vi "Transfer.vi"(7 "Timeout":i32 format="%d ms", 8 "error in":errorcluster, 9 "Parameters":T2 {"Data" format="%02x"; "Multiplexer"."Sub Index" format="%02x"; "Multiplexer"."Index" format="%04x"}, 10 "SDO Transfer":refnum<class "SDO Transfer.lvclass">, 11 "SDO Manager in":refnum<class "SDO Manager.lvclass">) -> (0 "error out":errorcluster, 3 "SDO Result":T3 {"SDO abort code"."Value" items=["Toggle bit not allowed"=84082688, "SDO protocol timed out"=84148224, "Client/server command specifier not valid or unknown"=84148225, "Invalid block size (block mode only)"=84148226, "Invalid sequence number (block mode only)"=84148227, "CRC error (block mode only)"=84148228, "Out of memory"=84148229, "Attempt to read a write only object"=100728833, "Attempt to write a read only object"=100728834, "Object does not exist in the object dictionary"=100794368, "Object cannot be mapped to the PDO"=100925505, "The number and length of the objects to be mapped would exceed PDO length"=100925506, "General parameter incompatibility reason"=100925507, "General internal incompatibility in the device"=100925511, "Access failed due to an hardware error"=101056512, "Data type does not match, length of service parameter does not match"=101122064, "Data type does not match, length of service parameter too high"=101122066, "Data type does not match, length of service parameter too low"=101122067, "Sub-index does not exist"=101253137, "Invalid value for parameter (download only)"=101253168, "Value of parameter written too high (download only)"=101253169, "Value of parameter written too low (download only)"=101253170, "Maximum value is less than minimum value"=101253174, "Resource not available: SDO connection"=101318691, "General error"=134217728, "Data cannot be transferred or stored to the application"=134217760, "Data cannot be transferred or stored to the application because of local control"=134217761, "Data cannot be transferred or stored to the application because of the present device stable"=134217762, "Object dictionary dynamic generation fails or no object dictionary is present (e.g. object dictionary is generated from file and generation fails because of an file error)"=134217763, "No data available"=134217764]; "Data"."Data" format="%02x"})   [LabVIEW 2020, in "SDO Manager.lvlib" / "SDO Manager.lvclass"]
uses:
  SDO Manager.lvclass
  SDO Transfer/SDO Transfer.lvclass
  SDO Manager.lvclass/SDO Manager.ctl
  SDO Transfer/SDO abort code.ctl
  Typedefs/SDO Result.ctl
  CANopen.lvlib
  Logging/Trace Type.ctl
  Logging/CANopen Logging.lvlib
  Logging/Log Level.vi
  Typedefs/Multiplexer.ctl
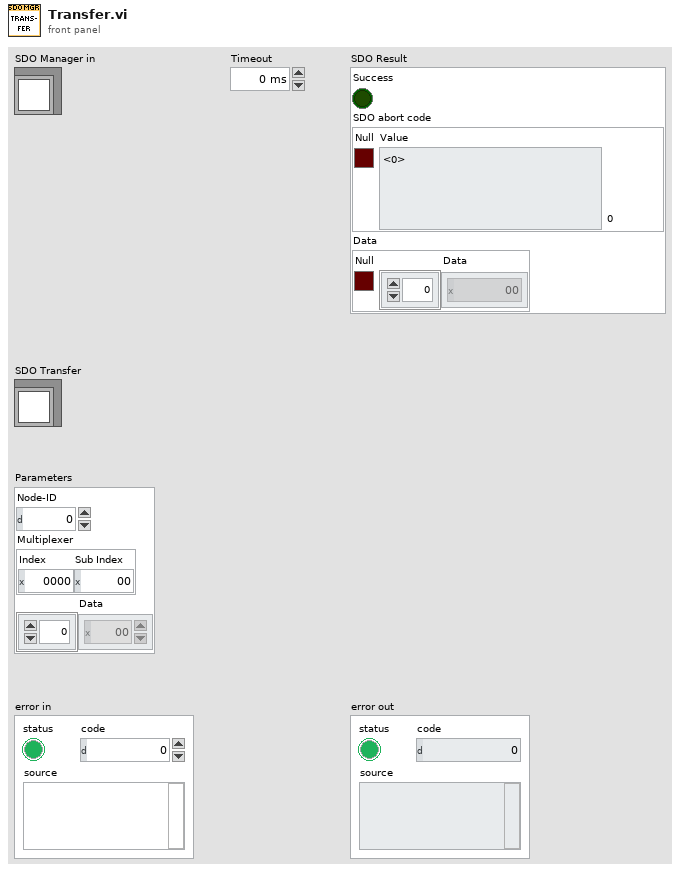
[diagram p1: front panel]
types:
  T1 = typedef "CANopen.lvlib/Multiplexer.ctl" = cluster{"Index":u16, "Sub Index":u8}
  T2 = cluster{"Node-ID":u8, "Multiplexer":T1, "Data":u8[]}
  T3 = typedef "CANopen.lvlib/SDO Result.ctl" = cluster{"Success":bool, "SDO abort code":cluster{"Null":bool, "Value":T4}, "Data":cluster{"Null":bool, "Data":u8[]}}
  T4 = typedef "SDO Manager.lvlib/SDO Transfer.lvclass/SDO abort code.ctl" = u32
  T5 = map{string, refnum<class "SDO Transfer.lvclass">}
  T6 = typedef "CANopen Logging.lvlib/Trace Type.ctl" = enum16{"Undefined", "Sent", "Received", "SDO Transfer"}
  T7 = enum16{"Error", "Warn", "Info", "Debug", "Trace"}
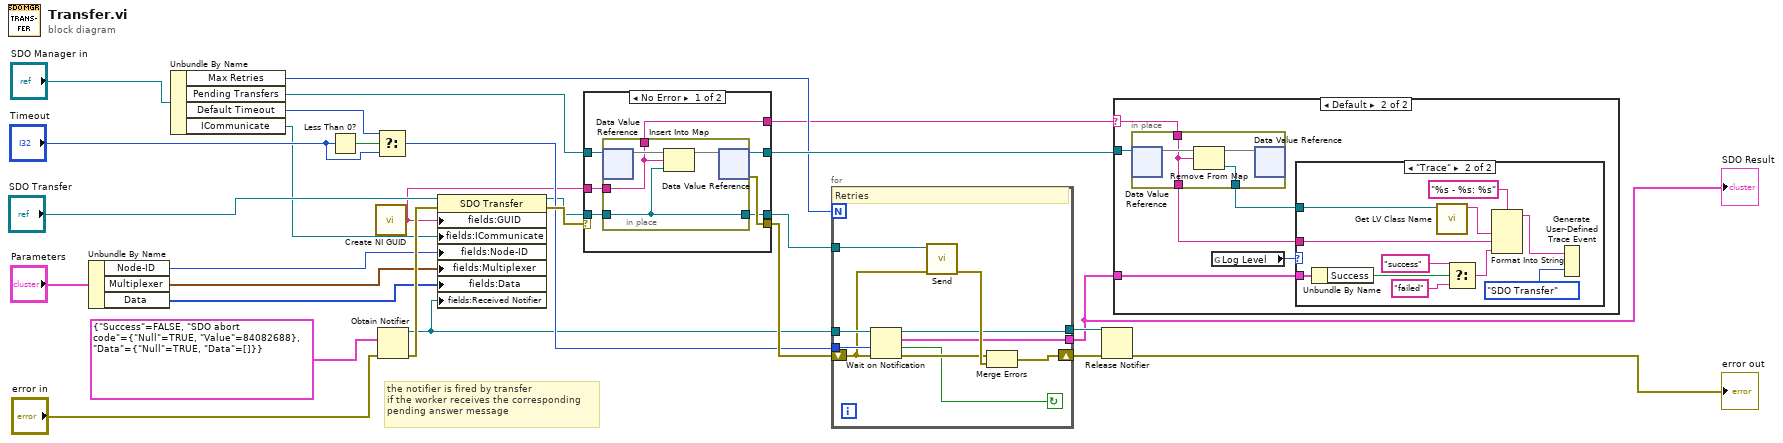
[diagram p0: block diagram]
diagram:
  # "the notifier is fired by transfer\nif the worker receives the corresponding\npending answer message"
  n1 = Unbundle By Name("Parameters") -> ("Node-ID"=w5:u8, "Multiplexer"=w7:T1, "Data"=w6:u8[])
  n2 = Unbundle By Name("SDO Manager in") -> ("Max Retries"=w23:u8, "Pending Transfers"=w22:refnum<data-value>, "Default Timeout"=w15:i32, "ICommunicate"=w4:refnum<class "ICommunicate.lvclass">)
  n3 = Less Than 0?(x="Timeout") -> (x < 0?=w14:bool)
  n4 = call <vilib>:"Create NI GUID.vi"() -> ("NI GUID"=w1:string)
  n5 = Select(t=w15, s=w14, f="Timeout") -> (s? t:f=w20:i32)
  n6 = Obtain Notifier(notification data type=T3 {"Success"=FALSE, "SDO abort code"={"Null"=TRUE, "Value"=84082688}, "Data"={"Null"=TRUE, "Data"=[]}}, error in (no error)="error in") -> (notifier out=w18:refnum<notifier>, error out=w19:errorcluster)  [unwired: 2 in, 1 out]
  n7 = property class="SDO Transfer"(reference="SDO Transfer", error in=w19, "fields:GUID"=w1, "fields:ICommunicate"=w4, "fields:Node-ID"=w5, "fields:Multiplexer"=w7, "fields:Data"=w6, "fields:Received Notifier"=w18) -> (reference out=w16:refnum<class "SDO Transfer.lvclass">, error out=w21:errorcluster)
  n8 = case shown="No Error" w21 {
    selector: w21 -> [_ w42]
    tunnel: w16 -> [w35 w41]
    tunnel: w22 -> [w34 w40]
    tunnel: [w33 w42] -> w25
    tunnel: [w32 w41] -> w24
    tunnel: [w31 w40] -> w27
    tunnel: [w30 _] -> w2
    tunnel: w1 -> [w29 _]
    frame No Error {
      n9 = in-place {
        in-place-border: w35 -> [w37]
        in-place-border: [w37] -> w32
        in-place-border: [w36] -> w30
        in-place-border: w29 -> [w36]
        n10 = in-place-dvr #1(w34) -> (w39:T5)  [unwired: 1 out]
        n11 = Insert Into Map(map in=w39, key=w36, value=w37) -> (map out=w38:T5)  [unwired: 2 out]
        n12 = in-place-dvr #1(w38) -> (w31:refnum<data-value>, w33:errorcluster)
      }
    }
    frame Error {
    }
  }
  n13 = for {
    N: w23 -> [_]
    tunnel: w18 -> [w52]
    tunnel: w20 -> [w51]
    tunnel: [w44] -> w3
    shift-right: [w48] -> w26
    shift-left: w25 -> [w49]
    tunnel: w24 -> [w50]
    tunnel: [w45] -> w28
    stop <- w43 continue-if-true
    # "Retries"
    n14 = Wait on Notification(notifier=w52, timeout in ms (-1)=w51, error in (no error)=w49) -> (notifier out=w45:refnum<notifier>, notification=w44:T3, timed out?=w43:bool, error out=w46:errorcluster)  [unwired: 1 in]
    n15 = call-dynamic "Send.vi"("error in"=w49, "SDO Transfer in"=w50) -> ("error out"=w47:errorcluster)  [unwired: 8 in, 1 out]
    n16 = Merge Errors(w46, w47) -> (w48:errorcluster)
  }
  "SDO Result" <- w3
  n17 = Release Notifier(notifier=w28, error in (no error)=w26) -> (error out=→"error out":errorcluster)  [unwired: 1 in, 2 out]
  n18 = case shown="Default" w2 {
    selector: w2 -> [_ w56]
    tunnel: w27 -> [_ w58]
    tunnel: w3 -> [_ w57]
    frame "" {
    }
    frame Default {
      n19 = in-place {
        in-place-border: w56 -> [w70]
        in-place-border: [w71] -> w55
        in-place-border: [w70] -> w54
        n20 = in-place-dvr #2(w58) -> (w73:T5)  [unwired: 1 out]
        n21 = Remove From Map(10:w70, 11:w73) -> (1:w71:refnum<class "SDO Transfer.lvclass">, 3:w72:T5)  [unwired: 1 out]
        n22 = in-place-dvr #2(w72) -> ()  [unwired: 2 out]
      }
      n23 = global read "Log Level.vi" "Log Level"() -> (w53:T7)
      n24 = case shown="\"Trace\"" w53 {
        tunnel: w57 -> [_ w69]
        tunnel: w55 -> [_ w62]
        tunnel: w54 -> [_ w61]
        frame Default {
        }
        frame "Trace" {
          n25 = Unbundle By Name(w69) -> ("Success"=w63:bool)
          n26 = call <vilib>:"Get LV Class Name.vi"("object"=w62) -> ("class name"=w65:string)  [unwired: 9 in, 1 out]
          n27 = Select(t="success", s=w63, f="failed") -> (s? t:f=w64:string)
          n28 = Format Into String(format string="%s - %s: %s" ("string"), w65, w61, w64) -> (resulting string=w67:string)  [unwired: 2 in, 1 out]
          n29 = Generate User-Defined Trace Event(1:Trace_Type."SDO Transfer" ("Trace Type"), 2:w67) -> ()
        }
      }
    }
  }
